vi "Keithley 2400 VSweep.vi"() -> ()   [LabVIEW 2020]
panel:
  in  "GPIB Address":refnum<visa-resource-name>="GPIB0::24::INSTR"
  in  "stop":bool
  in  "Step Size (mV)":dbl=50.0
  in  "Initial V":dbl format="%.2f"
  in  "HOLD LL":bool
  in  "HOLD UL":bool
  in  "Goto (V)":dbl format="%.3f"
  in  "UP Limit (V)":dbl=80.0 format="%.3f"
  in  "LW Limit (V)":dbl=-80.0 format="%.3f"
  in  "Sweep Rate UP (mV/s)":dbl=100.0
  in  "Sweep Rate DN (mV/s)":dbl=100.0
  out "Now at (V)":dbl format="%.3f"
  out "Status":enum16{"Sweep DN", "Sweep UP", "Fixed V"}(ring)
  in  "Sweep":bool=TRUE
  in  "Initialize Flag":bool
  out "Boolean":bool
  out "error out":T1
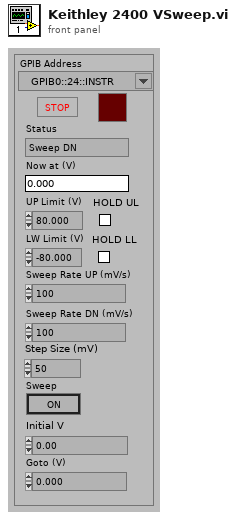
[diagram p1: front panel]
types:
  T1 = cluster{"error":bool, "code":i32, "source":string}
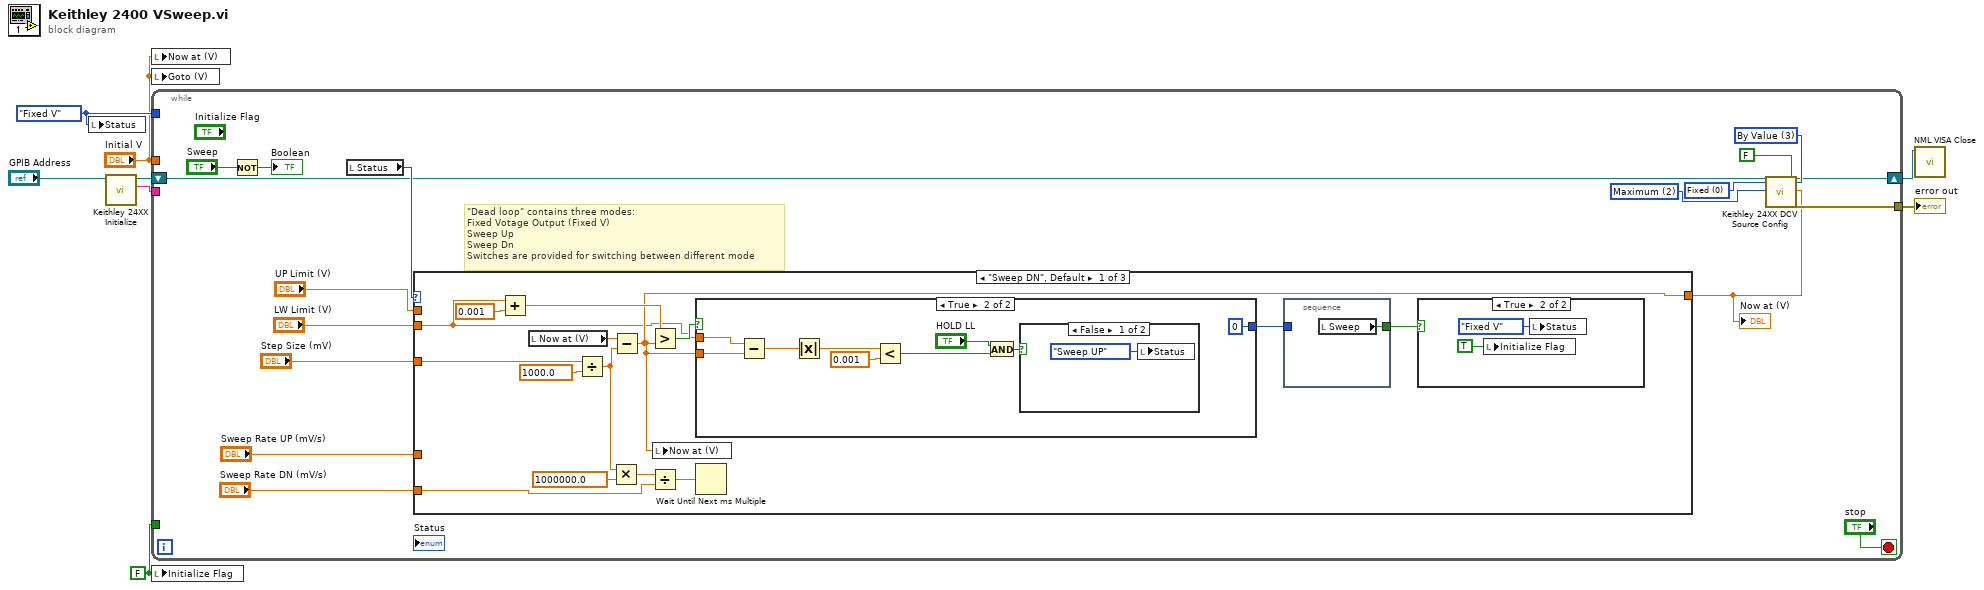
[diagram p0: block diagram]
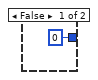
[diagram p3: hidden frame]
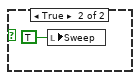
[diagram p4: hidden frame]
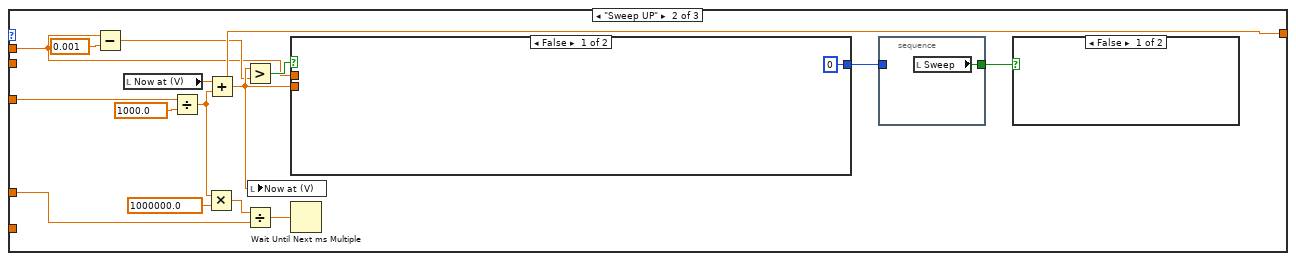
[diagram p5: hidden frame]
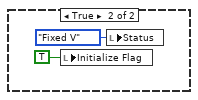
[diagram p6: hidden frame]
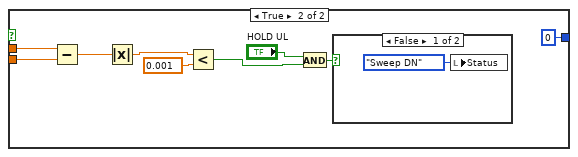
[diagram p7: hidden frame]
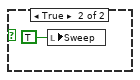
[diagram p8: hidden frame]
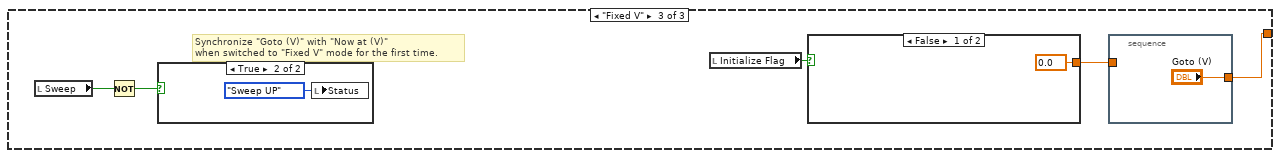
[diagram p9: hidden frame]
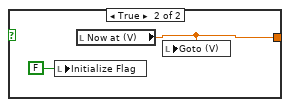
[diagram p10: hidden frame]
diagram:
  w5 = FALSE ("Initialize Flag")
  w6 = enum16{"Sweep DN", "Sweep UP", "Fixed V"}."Fixed V" ("Status")
  n1 = local write "Status"(w6) -> ()
  n2 = call "Keithley 24XX Initialize.vi"("GPIB Address"="GPIB Address") -> ("Instrument ID String"=w7:string, "dup VISA Session"=w2:refnum<visa-resource-name>)  [unwired: 4 in, 1 out]
  n3 = local write "Now at (V)"("Initial V") -> ()
  n4 = local write "Goto (V)"("Initial V") -> ()
  n5 = while {
    tunnel: [w17] -> w8
    tunnel: "Initial V" -> [_]
    tunnel: w7 -> [_]
    tunnel: w6 -> [_]
    tunnel: w5 -> [_]
    shift-right: [w9] -> w1
    shift-left: w2 -> [w10]
    stop <- "stop" stop-if-true
    w18 = u16 2 items=["Default 20V Range", "Minimum", "Maximum", "By Value", "Auto On", "Auto Off"] ("Range (Default:0)")
    w19 = u16 0 items=["Fixed", "Sweep", "List"] ("Mode Selection (Fixed:0)")
    w21 = u16 3 items=["Default 0V", "Minimum", "Maximum", "By Value"] ("Level (Default:0)")
    # "\"Dead loop\" contains three modes:\nFixed Votage Output (Fixed V)\nSweep Up\nSweep Dn\nSwitches are provided for switching between different mode"
    n6 = Not(x="Sweep") -> (.not. x?=→"Boolean":bool)
    n7 = local read "Status"() -> (w16:enum16{"Sweep DN", "Sweep UP", "Fixed V"})
    n8 = case shown="\"Sweep DN\", Default" w16 {
      tunnel: "Sweep Rate UP (mV/s)" -> [_ w66 _]
      tunnel: "UP Limit (V)" -> [_ w56 _]
      tunnel: "LW Limit (V)" -> [w26 _ _]
      tunnel: "Sweep Rate DN (mV/s)" -> [w38 _ _]
      tunnel: [w27 w59 w90] -> w12
      tunnel: "Step Size (mV)" -> [w33 w61 _]
      frame "Sweep DN", Default {
        n9 = Add(x=w26, y=0.001) -> (x+y=w28:dbl)
        n10 = local read "Now at (V)"() -> (w40:dbl)
        n11 = Divide(x=w33, y=1000.0) -> (x/y=w31:dbl)
        n12 = Multiply(x=w31, y=1000000.0) -> (x*y=w39:dbl)
        n13 = Subtract(x=w40, y=w31) -> (x-y=w27:dbl)
        n14 = Greater?(x=w28, y=w27) -> (0:w36:bool)
        n15 = Divide(x=w39, y=w38) -> (x/y=w37:dbl)
        n16 = local write "Now at (V)"(w27) -> ()
        n17 = case shown="True" w36 {
          tunnel: [0 0] -> w30
          tunnel: w27 -> [_ w51]
          tunnel: w26 -> [_ w52]
          frame False {
          }
          frame True {
            n18 = Subtract(x=w52, y=w51) -> (x-y=w50:dbl)
            n19 = Absolute Value(x=w50) -> (abs(x)=w49:dbl)
            n20 = Less?(x=w49, y=0.001) -> (x < y?=w45:bool)
            n21 = And(x="HOLD LL", y=w45) -> (x .and. y?=w47:bool)
            n22 = case shown="False" w47 {
              frame False {
                n23 = local write "Status"(enum16{"Sweep DN", "Sweep UP", "Fixed V"}."Sweep UP" ("Status")) -> ()
              }
              frame True {
                n24 = local write "Sweep"(TRUE ("Sweep")) -> ()
              }
            }
          }
        }
        n25 = Wait Until Next ms Multiple(millisecond multiple=w37) -> ()  [unwired: 1 out]
        n26 = stacked-sequence {
          tunnel: [w41] -> w35
          tunnel: w30 -> [_]
          frame #0 {
            n27 = local read "Sweep"() -> (w41:bool)
          }
        }
        n28 = case shown="True" w35 {
          frame False {
          }
          frame True {
            n29 = local write "Initialize Flag"(TRUE ("Initialize Flag")) -> ()
            n30 = local write "Status"(enum16{"Sweep DN", "Sweep UP", "Fixed V"}."Fixed V" ("Status")) -> ()
          }
        }
      }
      frame "Sweep UP" {
        n31 = Subtract(x=w56, y=0.001) -> (x-y=w57:dbl)
        n32 = local read "Now at (V)"() -> (w70:dbl)
        n33 = Divide(x=w61, y=1000.0) -> (x/y=w62:dbl)
        n34 = Multiply(x=w62, y=1000000.0) -> (x*y=w68:dbl)
        n35 = Add(x=w70, y=w62) -> (x+y=w59:dbl)
        n36 = Greater?(x=w59, y=w57) -> (0:w65:bool)
        n37 = Divide(x=w68, y=w66) -> (x/y=w69:dbl)
        n38 = local write "Now at (V)"(w59) -> ()
        n39 = case shown="False" w65 {
          tunnel: [0 0] -> w60
          tunnel: w56 -> [_ w82]
          tunnel: w59 -> [_ w81]
          frame False {
          }
          frame True {
            n40 = Subtract(x=w82, y=w81) -> (x-y=w78:dbl)
            n41 = Absolute Value(x=w78) -> (abs(x)=w77:dbl)
            n42 = Less?(x=w77, y=0.001) -> (x < y?=w75:bool)
            n43 = And(x="HOLD UL", y=w75) -> (x .and. y?=w80:bool)
            n44 = case shown="False" w80 {
              frame False {
                n45 = local write "Status"(enum16{"Sweep DN", "Sweep UP", "Fixed V"}."Sweep DN" ("Status")) -> ()
              }
              frame True {
                n46 = local write "Sweep"(TRUE ("Sweep")) -> ()
              }
            }
          }
        }
        n47 = Wait Until Next ms Multiple(millisecond multiple=w69) -> ()  [unwired: 1 out]
        n48 = stacked-sequence {
          tunnel: [w71] -> w64
          tunnel: w60 -> [_]
          frame #0 {
            n49 = local read "Sweep"() -> (w71:bool)
          }
        }
        n50 = case shown="False" w64 {
          frame False {
          }
          frame True {
            n51 = local write "Initialize Flag"(TRUE ("Initialize Flag")) -> ()
            n52 = local write "Status"(enum16{"Sweep DN", "Sweep UP", "Fixed V"}."Fixed V" ("Status")) -> ()
          }
        }
      }
      frame "Fixed V" {
        # "Synchronize \"Goto (V)\" with \"Now at (V)\"\nwhen switched to \"Fixed V\" mode for the first time."
        n53 = local read "Sweep"() -> (w87:bool)
        n54 = Not(x=w87) -> (.not. x?=w86:bool)
        n55 = case shown="True" w86 {
          frame False {
          }
          frame True {
            n56 = local write "Status"(enum16{"Sweep DN", "Sweep UP", "Fixed V"}."Sweep UP" ("Status")) -> ()
          }
        }
        n57 = local read "Initialize Flag"() -> (w89:bool)
        n58 = case shown="False" w89 {
          tunnel: [0.0 ("Now at  (V)") w92] -> w88
          frame False {
          }
          frame True {
            n59 = local write "Initialize Flag"(FALSE ("Initialize Flag")) -> ()
            n60 = local read "Now at (V)"() -> (w92:dbl)
            n61 = local write "Goto (V)"(w92) -> ()
          }
        }
        n62 = stacked-sequence {
          tunnel: ["Goto (V)"] -> w90
          tunnel: w88 -> [_]
          frame #0 {
          }
        }
      }
    }
    "Now at (V)" <- w12
    n63 = call "Keithley 24XX DCV Source Config.vi"("VISA resource name"=w10, "Mode Selection (Fixed:0)"=w19, "Range (Default:0)"=w18, "Output Mode"=FALSE, "Level (Default:0)"=w21, "Output Value (Volts)"=w12) -> ("dup VISA Session"=w9:refnum<visa-resource-name>, "error out"=w17:T1)  [unwired: 20 in]
  }
  "error out" <- w8
  n64 = local write "Initialize Flag"(w5) -> ()
  n65 = call "NML VISA Close.vi"("VISA resource name"=w1) -> ()  [unwired: 10 in, 1 out]
